vi "HFRR ADV v015 new software.vi"() -> ()   [LabVIEW 2025] (continued)
              frame False {
              }
              frame True {
                n2567 = local write "Rt 3"(FALSE ("Rt 3")) -> ()
                n2568 = local write "Json End Flg"(TRUE ("Upld AR 2")) -> ()
              }
            }
            "Rt" <- TRUE ("Rt")
            "Rt 2" <- FALSE ("Rt")
          }
          frame True {
            n2569 = local read "Rt"() -> (w3002:bool)
            n2570 = local write "Rt 2"(TRUE ("Rt 2")) -> ()
            n2571 = case shown="True" w3002 {
              frame False {
              }
              frame True {
                w3003 = TRUE ("Upld AR 2")
                n2572 = local write "Rt"(FALSE ("Rt")) -> ()
                n2573 = local write "Upld AR"(w3003) -> ()
                n2574 = local write "Json St Flg"(w3003) -> ()
              }
            }
            "Rt 3" <- TRUE ("Rt 3")
          }
        }
        n2575 = case shown="True" w2853 {
          tunnel: [FALSE ("RUN") TRUE ("RUN")] -> w2852
          tunnel: [_ 2] -> w2846
          frame False {
          }
          frame True {
          }
        }
        n2576 = case shown="True" w2851 {
          tunnel: [FALSE ("RUN") TRUE ("RUN")] -> w2850
          tunnel: [_ 3] -> w2845
          frame False {
          }
          frame True {
          }
        }
        n2577 = case shown="\"Acquire\"" w2831 {
          tunnel: w2833 -> [_ w3064]
          frame Default {
            w3063 = 0.0 ("output")
            n2578 = local write "PID-out"(w3063) -> ()
            n2579 = local write "Frequency ( Hz )"(w3063) -> ()
          }
          frame "Acquire" {
            n2580 = stacked-sequence {
              frame #0 {
                n2581 = local read "Auto Start Test"() -> (w3066:bool)
                n2582 = case shown="True" w3066 {
                  tunnel: "RUN" -> [w3087 w3090]
                  tunnel: [w3087 w3089] -> w3067
                  frame False {
                  }
                  frame True {
                    n2583 = local read "Auto Start Temp"() -> (w3088:bool)
                    n2584 = Or(x=w3090, y=w3088) -> (x .or. y?=w3089:bool)
                  }
                }
                n2585 = local read "clk"() -> (w3086:dbl)
                n2586 = local read "Save"() -> (w3082:bool)
                n2587 = Equal?(x=w3086, y=0.0) -> (x = y?=w3083:bool)
                n2588 = And(x=w3083, y=w3082) -> (x .and. y?=w3084:bool)
                n2589 = Not(x="Engage") -> (.not. x?=w3073:bool)
                n2590 = case shown="False" w3067 {
                  tunnel: [0.0 w3113] -> w3069
                  frame False {
                    (unwired) TRUE ("Visible")
                    n2591 = local read "Auto Start Test"() -> (w3094:bool)
                    n2592 = local write "Start Time"(TRUE ("Start Time")) -> ()
                    n2593 = property on="Stroke 2" class="DigNum (strict)"("Visible"=FALSE) -> ()  [unwired: 2 in, 2 out]
                    n2594 = case shown="False" w3094 {
                      frame False {
                        n2595 = property on="Heater Button" class="Bool (strict)"("DisabledEnum"=T18."Enabled" ("Disabled")) -> ()  [unwired: 2 in, 2 out]
                        n2596 = property on="Humidity" class="Bool (strict)"("DisabledEnum"=T18."Enabled" ("Disabled")) -> ()  [unwired: 2 in, 2 out]
                      }
                      frame True {
                      }
                    }
                    n2597 = case shown="False" "TestCompFlg" {
                      frame False {
                        n2598 = local read "StartFlg"() -> (w3102:bool)
                        n2599 = case shown="True" w3102 {
                          frame False {
                          }
                          frame True {
                            n2600 = stacked-sequence {
                              frame #0 {
                                n2601 = local read "EVENT LOG"() -> (w3106:string)
                                n2602 = call "Event Log.vi"("Content"="Test was interrupted", "EVENT LOG"=w3106) -> ("EVENT LOG"=w3107:string)  [unwired: 8 in, 1 out]
                                n2603 = local write "EVENT LOG"(w3107) -> ()
                                n2604 = property on="RUN" class="Bool (strict)"("Visible"=TRUE) -> ()  [unwired: 2 in, 2 out]
                                n2605 = property on="Auto Start Test" class="Bool (strict)"("Visible"=TRUE) -> ()  [unwired: 2 in, 2 out]
                              }
                              frame #1 {
                                w3109 = FALSE ("StartFlg")
                                n2606 = property on="Heater Button" class="Bool (strict)"("Val(Sgnl)"=FALSE ("Value (Signaling)")) -> ()  [unwired: 2 in, 2 out]
                                n2607 = local write "Heater Button"(w3109) -> ()
                                n2608 = local write "StartFlg"(w3109) -> ()
                                n2609 = local write "Humidity"(w3109) -> ()
                              }
                              frame #2 {
                                n2610 = local write "Command"("VC;0" ("Command")) -> ()
                              }
                              frame #3 {
                                n2611 = Wait (ms)(milliseconds to wait=u32 1500) -> ()  [unwired: 1 out]
                              }
                              frame #4 {
                                n2612 = local write "Command"("HE;0" ("Command")) -> ()
                              }
                            }
                          }
                        }
                      }
                      frame True {
                      }
                    }
                    n2613 = local write "String 14"("Test will autostart once parameters reach the set value." ("String 14")) -> ()
                  }
                  frame True {
                    (unwired) FALSE ("Visible")
                    n2614 = property on="Stroke 2" class="DigNum (strict)"("Visible"=TRUE) -> ()  [unwired: 2 in, 2 out]
                    n2615 = property on="STOP 2" class="Bool (strict)"("Disabled"=u8 2) -> ()  [unwired: 2 in, 2 out]
                    n2616 = local write "String 14"(" Running....." ("String 14")) -> ()
                    n2617 = property on="Heater Button" class="Bool (strict)"("DisabledEnum"=T18."Disabled and Grayed Out" ("Disabled")) -> ()  [unwired: 2 in, 2 out]
                    n2618 = property on="Humidity" class="Bool (strict)"("DisabledEnum"=T18."Disabled and Grayed Out" ("Disabled")) -> ()  [unwired: 2 in, 2 out]
                    n2619 = case shown="True" "Start Time" {
                      selector: "Start Time" -> [_ w3132]
                      frame False {
                      }
                      frame True {
                        n2620 = Not(x=w3132) -> (.not. x?=w3131:bool)
                        n2621 = local write "Start Time"(w3131) -> ()
                        n2622 = local read "EVENT LOG"() -> (w3133:string)
                        n2623 = call "Event Log.vi"("Content"="Test in progress", "EVENT LOG"=w3133) -> ("EVENT LOG"=w3135:string)  [unwired: 8 in, 1 out]
                        n2624 = local write "EVENT LOG"(w3135) -> ()
                      }
                    }
                    n2625 = disable-structure shown="Enabled" {
                      disable-tunnel: [w3124 w3130] -> w3113
                      frame Disabled {
                        n2626 = local read "Set Hz"() -> (w3127:dbl)
                        n2627 = call <vilib>:"Uniform White Noise Waveform.vi"() -> ("signal out"=w3126:waveform(dbl))  [unwired: 10 in, 1 out]
                        n2628 = Random Number (0-1)() -> (number: 0 to 1=w3123:dbl)
                        n2629 = Add(x=w3127, y=w3126) -> (x+y=w3125:waveform(dbl))
                        n2630 = Multiply(x=ext 0.01 ("y"), y=w3123) -> (x*y=w3121:ext)
                        n2631 = Multiply(x=w3125, y=w3121) -> (x*y=w3124:waveform(ext))
                      }
                      frame Enabled {
                        n2632 = call-poly <vilib>:"Random Number (Range).vi"("lower bound (0)"=49.89, "upper bound (100)"=50.8) -> ("number"=w3130:dbl)  [unwired: 9 in]
                      }
                    }
                    "StartFlg" <- TRUE ("StartFlg")
                  }
                }
                n2633 = case shown="True" w3084 {
                  frame False {
                  }
                  frame True {
                    n2634 = local write "clk"(10.0 ("clk")) -> ()
                    n2635 = Get Date/Time In Seconds() -> (seconds since 1Jan1904=w3138:timestamp)
                    n2636 = To Double Precision Float(number=w3138) -> (double precision float=w3136:dbl)
                    n2637 = local write "acq timer"(w3136) -> ()
                    n2638 = local write "act save time"(w3136) -> ()
                  }
                }
                n2639 = call "Elapsed Time"("Time Target (s)"="Countdown", "Reset"=w3073) -> ("Elapsed Time (s)"=w3078:dbl, "Time has Elapsed"=w3076:bool)  [unwired: 10 in, 6 out]
                "Countdown 2" <- w3078
                n2640 = Subtract(x=w3078, y=2.0) -> (x-y=w3081:dbl)
                n2641 = Less?(x=w3081, y="Countdown") -> (x < y?=w3079:bool)
                n2642 = And(x=w3079, y=w3076) -> (x .and. y?=w3075:bool)
                n2643 = case shown="True" w3075 {
                  frame False {
                  }
                  frame True {
                    (unwired) dbl[] [] ("History Data")
                    n2644 = local write "Engage"(FALSE ("Engage")) -> ()
                    n2645 = local write "RUN"(TRUE ("RUN")) -> ()
                    n2646 = local read "Humidity ( %RH )"() -> (→"Rh Before":dbl)
                  }
                }
                n2647 = local read "Test \nStatus"() -> (w3071:bool)
                n2648 = Select(t=w3069, s=w3071, f=0.0) -> (s? t:f=w3070:dbl)
                n2649 = local write "Frequency ( Hz )"(w3070) -> ()
              }
              frame #1 {
                w3161 = 1000000.0 ("x")
                # "HC;1/0\nST;VALUE"
                # "Elapsed time\ncof\nstroke\nAir temp\nTemp\nHumidity"
                # "acq timer\n\nact save time"
                # "convert to microseconds"
                n2650 = local read "COUNT"() -> (w3144:i32)
                n2651 = local read "Rate"() -> (w3157:dbl)
                n2652 = Divide(x=w3161, y=w3157) -> (x/y=w3162:dbl)
                n2653 = Greater Or Equal?(x=w3144, y=250) -> (x >= y?=w3143:bool)
                n2654 = Get Date/Time In Seconds() -> (seconds since 1Jan1904=w3164:timestamp)
                n2655 = case shown="True" w3143 {
                  frame False {
                    n2656 = local read "COUNT"() -> (w3165:i32)
                    n2657 = Increment(x=w3165) -> (x+1=w3166:i32)
                    n2658 = local write "COUNT"(w3166) -> ()
                  }
                  frame True {
                    n2659 = local write "COUNT"(0 ("COUNT")) -> ()
                  }
                }
                n2660 = local read "Samplingtime 2"() -> (w3142:dbl)
                n2661 = local read "act save time"() -> (w3159:dbl)
                n2662 = Divide(x=w3162, y=w3161) -> (x/y=w3160:dbl)
                n2663 = To Double Precision Float(number=w3164) -> (double precision float=w3153:dbl)
                n2664 = Add(x=w3159, y=w3142) -> (x+y=w3158:dbl)
                n2665 = local read "acq timer"() -> (w3163:dbl)
                n2666 = local read "COUNT"() -> (w3146:i32)
                n2667 = Greater Or Equal?(x=w3153, y=w3158) -> (x >= y?=w3141:bool)
                n2668 = Multiply(x=w3160, y=w3146) -> (x*y=w3152:dbl)
                n2669 = Subtract(x=w3153, y=w3163) -> (x-y=w3155:dbl)
                n2670 = local read "Save"() -> (w3156:bool)
                n2671 = Add(x=w3155, y=w3152) -> (x+y=w3139:dbl)
                "Elapsed time 3" <- w3139
                n2672 = And(x=w3141, y=w3156) -> (x .and. y?=w3154:bool)
                n2673 = Divide(x=w3139, y=60.0) -> (x/y=w3150:dbl)
                n2674 = local read "Test \nStatus"() -> (w3140:bool)
                n2675 = local read "clk"() -> (w3147:dbl)
                n2676 = Equal?(x=w3147, y=10.0) -> (x = y?=w3149:bool)
                n2677 = case shown="True" w3154 {
                  tunnel: w3153 -> [_ w3277]
                  tunnel: [FALSE ("Boolean 2") TRUE ("Boolean 2")] -> _
                  frame False {
                  }
                  frame True {
                    w3231 = ";" ("Substring")
                    # "Pid out/\nFreq response value"
                    n2678 = local write "act save time"(w3277) -> ()
                    n2679 = local read "FILE"() -> (w3225:string)
                    n2680 = call "file check.vi"("file name in"=w3225) -> ("error out"=w3228:errorcluster, "file name out"=w3223:string)  [unwired: 9 in]
                    n2681 = local read "LVDT STROKE"() -> (w3220:dbl)
                    n2682 = local read "Add up Stroke"() -> (w3218:dbl)
                    n2683 = call "FILE PATH CREATION.vi"("error in"=w3228, "FILE NAME :"=w3223) -> ("FILE OUT"=w3226:path)  [unwired: 8 in, 1 out]
                    n2684 = Concatenate Strings(w3223, ".dgf" ("Substring")) -> (w3227:string)
                    n2685 = Subtract(x=w3220, y=w3218) -> (x-y=w3219:dbl)
                    n2686 = Absolute Value(x=w3219) -> (abs(x)=w3217:dbl)
                    n2687 = local read "FF 2"() -> (→"Frictional Force ( N )" →"Frictional Force ( N )":dbl)
                    n2688 = Build Path(base path=w3226, name or relative path=w3227) -> (appended path=w3222:path)
                    n2689 = local read "COF 2"() -> (w3236:dbl)
                    "cof" <- w3236
                    "Coefficient of Friction" <- w3236
                    "COF 4" <- w3236
                    "Coefficient of Friction" <- w3236
                    n2690 = local read "TEMP"() -> (w3239:dbl)
                    "Temp" <- w3239
                    "Temperature ( Deg C )" <- w3239
                    n2691 = local read "Humidity ( %RH )"() -> (w3238:dbl)
                    "Humidity ( %RH )" <- w3238
                    "Humidity ( %RH )" <- w3238
                    n2692 = local read "Frequency ( Hz )"() -> (w3245:dbl)
                    n2693 = call <vilib>:"Mean PtByPt.vi"("x"=w3217, "sample length"="STROKE FILTER") -> ("mean"=w3216:dbl)  [unwired: 2 in, 1 out]
                    n2694 = local read "Elapsed time"() -> (w3270:dbl)
                    n2695 = local read "AIR TEMP"() -> (w3243:dbl)
                    n2696 = local read "PID-out"() -> (w3248:dbl)
                    n2697 = local write "Temperature ( Deg C )"(w3239) -> ()
                    n2698 = Number To Fractional String(number=w3216, width (-)=i16 9 ("precision (6)"), precision (6)=i16 6) -> (F-format string=w3263:string)  [unwired: 1 in]
                    n2699 = Number To Fractional String(number=w3243, width (-)=i16 9 ("precision (6)"), precision (6)=i16 3) -> (F-format string=w3262:string)  [unwired: 1 in]
                    n2700 = Number To Fractional String(number=w3239, width (-)=i16 9 ("precision (6)"), precision (6)=i16 3) -> (F-format string=w3259:string)  [unwired: 1 in]
                    n2701 = Number To Fractional String(number=w3238, width (-)=i16 9 ("precision (6)"), precision (6)=i16 3) -> (F-format string=w3256:string)  [unwired: 1 in]
                    n2702 = Number To Fractional String(number=0.0, width (-)=i16 9 ("precision (6)"), precision (6)=i16 3) -> (F-format string=w3253:string)  [unwired: 1 in]
                    n2703 = Number To Fractional String(number=w3248, width (-)=i16 9 ("precision (6)"), precision (6)=i16 3) -> (F-format string=w3249:string)  [unwired: 1 in]
                    n2704 = Number To Fractional String(number=w3245, width (-)=i16 9 ("precision (6)"), precision (6)=i16 3) -> (F-format string=w3244:string)  [unwired: 1 in]
                    n2705 = Number To Fractional String(number=w3236, width (-)=i16 9 ("precision (6)"), precision (6)=i16 6) -> (F-format string=w3271:string)  [unwired: 1 in]
                    n2706 = Number To Fractional String(number=w3270, width (-)=i16 14 ("precision (6)"), precision (6)=i16 3) -> (F-format string=w3272:string)  [unwired: 1 in]
                    n2707 = Bundle("y"=1.02, "mean"=w3216, "y"=0.98) -> (w3237:cluster{"y":dbl, "mean":dbl, "y":dbl})  [unwired: 1 in]
                    n2708 = Number To Fractional String(number="Ambient Humidity :", width (-)=i16 9 ("precision (6)"), precision (6)=i16 6) -> (F-format string=w3229:string)  [unwired: 1 in]
                    n2709 = local read "RUN"() -> (w3235:bool)
                    n2710 = case shown="True" w3235 {
                      tunnel: w3237 -> [_ w3282]
                      tunnel: w3216 -> [_ w3281]
                      tunnel: w3216 -> [_ w3279]
                      tunnel: w3216 -> [_ w3280]
                      frame False {
                      }
                      frame True {
                        "Stroke ( mm )" <- w3282
                        "Stroke ( mm )" <- w3282
                        "Stroke 4" <- w3281
                        "Stroke 3" <- w3279
                        "Stroke 2" <- w3280
                        "measured_stroke" <- w3279
                      }
                    }
                    n2711 = Concatenate Strings(w3272, w3231, w3271, w3231, w3263, w3231, w3262, w3231, w3259, w3231, w3256, w3231, w3253, w3231, w3249, w3231, w3244, w3231, w3229, "\r") -> (w3269:string)
                    n2712 = call <vilib>:"Write Characters To File.vi"("append to file? (new file:F)"=TRUE, "character string"=w3269, "file path (dialog if empty)"=w3222) -> ()  [unwired: 2 in, 1 out]
                    "refresh flag" <- TRUE ("refresh flag")
                  }
                }
                n2713 = case shown="True" w3140 {
                  tunnel: w3150 -> [_ w3176]
                  tunnel: w3155 -> [_ w3186]
                  tunnel: [0.0 w3182] -> _
                  tunnel: w3149 -> [_ w3181]
                  tunnel: [0.0 w3180] -> _
                  tunnel: w3139 -> [_ w3180]
                  tunnel: w3153 -> [w3169 _]
                  frame False {
                    n2714 = local write "acq timer"(w3169) -> ()
                    n2715 = local write "Test Duration Status"(0.0 ("Test Duration Status")) -> ()
                  }
                  frame True {
                    n2716 = local read "Set Hz"() -> (w3183:dbl)
                    n2717 = local write "Elapsed time"(w3176) -> ()
                    n2718 = local read "test time"() -> (w3175:dbl)
                    n2719 = Multiply(x=w3186, y=w3183) -> (x*y=w3185:dbl)
                    n2720 = case shown="False" w3181 {
                      tunnel: w3185 -> [w3187 _]
                      tunnel: [w3187 1.0] -> w3182
                      frame False {
                        n2721 = local write "Cycles elapsed"(w3187) -> ()
                      }
                      frame True {
                      }
                    }
                    n2722 = Greater?(x=w3176, y=w3175) -> (0:w3184:bool)
                    n2723 = Subtract(x=w3175, y=w3176) -> (x-y=w3174:dbl)
                    "time" <- w3174
                    n2724 = Multiply(x=w3174, y=60.0) -> (x*y=w3173:dbl)
                    n2725 = local write "Time Remaining"(w3173) -> ()
                    n2726 = local write "Remaining Time"(w3173) -> ()
                    n2727 = case shown="True" w3184 {
                      frame False {
                      }
                      frame True {
                        n2728 = stacked-sequence {
                          frame #0 {
                            w3192 = T18."Enabled" ("Disabled")
                            w3191 = FALSE ("TEST FILE NAM,E SAVED")
                            w3193 = "" ("FILE")
                            w3194 = TRUE ("Visible")
                            n2729 = local write "Humidity"(FALSE ("Humidity")) -> ()
                            n2730 = local write "RUN"(FALSE ("OK Button 2")) -> ()
                            n2731 = local write "Heater Button"(FALSE ("Heater Button")) -> ()
                            n2732 = local write "Auto Start Test"(FALSE ("Auto Start Test")) -> ()
                            n2733 = local write "TestCompFlg"(TRUE ("StpFlg")) -> ()
                            n2734 = local read "Humidity ( %RH )"() -> (→"Rh After":dbl)
                            n2735 = property on="STOP 2" class="Bool (strict)"("Disabled"=u8 0) -> ()  [unwired: 2 in, 2 out]
                            n2736 = local read "EVENT LOG"() -> (w3199:string)
                            n2737 = call "Event Log.vi"("Content"="Test Completed", "EVENT LOG"=w3199) -> ("EVENT LOG"=w3198:string)  [unwired: 8 in, 1 out]
                            n2738 = property on="RUN" class="Bool (strict)"("Visible"=w3194) -> ()  [unwired: 2 in, 2 out]
                            n2739 = property on="Auto Start Test" class="Bool (strict)"("Visible"=w3194) -> ()  [unwired: 2 in, 2 out]
                            n2740 = local write "Batch Ref Num :"(w3193) -> ()
                            n2741 = local write "FILE"(w3193) -> ()
                            n2742 = local write "EVENT LOG"(w3198) -> ()
                            n2743 = local write "TEST FILE NAM,E SAVED"(w3191) -> ()
                            n2744 = local write "Fuel Discription :"(w3193) -> ()
                            n2745 = local write "START TEMP"(w3191) -> ()
                            n2746 = local write "Remarks :"(w3193) -> ()
                            n2747 = local write "Main Dashboard Buttons"(T1."Imaging" ("Main Dashboard Buttons")) -> ()
                            n2748 = local write "Main Tab"(T2."Adv Scar" ("Main Tab")) -> ()
                            n2749 = property on="FRICVALZ 2" class="Bool (strict)"("DisabledEnum"=w3192) -> ()  [unwired: 2 in, 2 out]
                            n2750 = property on="FRICVALZ 3" class="Bool (strict)"("DisabledEnum"=w3192) -> ()  [unwired: 2 in, 2 out]
                            n2751 = property on="FRICVALZ 4" class="Bool (strict)"("DisabledEnum"=w3192) -> ()  [unwired: 2 in, 2 out]
                          }
                          frame #1 {
                            n2752 = Wait (ms)(milliseconds to wait=u32 1500) -> ()  [unwired: 1 out]
                          }
                          frame #2 {
                            n2753 = local write "Command"("VC;0") -> ()
                          }
                          frame #3 {
                            n2754 = Wait (ms)(milliseconds to wait=u32 1500) -> ()  [unwired: 1 out]
                          }
                          frame #4 {
                            n2755 = local write "Command"("VC;0") -> ()
                          }
                          frame #5 {
                            n2756 = Wait (ms)(milliseconds to wait=u32 1500) -> ()  [unwired: 1 out]
                          }
                          frame #6 {
                            n2757 = local write "Command"("ST;0") -> ()
                          }
                          frame #7 {
                            n2758 = local write "measured_stroke"(0.0 ("measured_stroke")) -> ()
                            n2759 = Wait (ms)(milliseconds to wait=u32 1500) -> ()  [unwired: 1 out]
                          }
                          frame #8 {
                            n2760 = local write "Command"("HE;0") -> ()
                          }
                        }
                      }
                    }
                    n2761 = Divide(x=w3176, y=w3175) -> (x/y=w3179:dbl)
                    n2762 = Multiply(x=w3179, y=100.0) -> (x*y=w3177:dbl)
                    n2763 = local write "Test Duration Status"(w3177) -> ()
                  }
                }
              }
              frame #2 {
                n2764 = case shown="True" "Heater Button" {
                  tunnel: [0.0 ("output") w3305] -> w3283
                  frame False {
                    w3286 = TRUE ("tmpchk")
                    n2765 = local read "TEMP"() -> (w3287:dbl)
                    n2766 = local write "Temp ini"(w3287) -> ()
                    n2767 = local write "Reset 4"(w3286) -> ()
                    n2768 = local write "tmpchk"(w3286) -> ()
                    n2769 = local write "reinit"(TRUE ("reinit")) -> ()
                    n2770 = local write "manual temp log"(TRUE ("manual temp log")) -> ()
                  }
                  frame True {
                    # "Logic to turn off\nthe heater when \ntemp is not rising.\nTime - 60 sec\nDelta t- 5°c"
                    n2771 = local read "Temp ini"() -> (w3294:dbl)
                    n2772 = local read "Auto Start Test"() -> (w3290:bool)
                    n2773 = Less?(x=w3294, y=53.0) -> (x < y?=w3292:bool)
                    n2774 = case shown="False" w3290 {
                      frame False {
                        n2775 = local read "Set Temp"() -> (w3314:dbl)
                        n2776 = local read "TEMP"() -> (w3313:dbl)
                        n2777 = Subtract(x=w3314, y=w3313) -> (x-y=w3312:dbl)
                        n2778 = Absolute Value(x=w3312) -> (abs(x)=w3311:dbl)
                        n2779 = Less?(x=w3311, y=0.5) -> (x < y?=w3309:bool)
                        n2780 = case shown="True" w3309 {
                          tunnel: "manual temp log" -> [_ w3315]
                          frame False {
                          }
                          frame True {
                            n2781 = case shown="True" w3315 {
                              selector: w3315 -> [_ w3316]
                              frame False {
                              }
                              frame True {
                                # "#Event log"
                                n2782 = Not(x=w3316) -> (.not. x?=w3317:bool)
                                n2783 = local write "manual temp log"(w3317) -> ()
                                n2784 = local read "EVENT LOG"() -> (w3320:string)
                                n2785 = call "Event Log.vi"("Content"="Target Temperature reached", "EVENT LOG"=w3320) -> ("EVENT LOG"=w3319:string)  [unwired: 8 in, 1 out]
                                n2786 = local write "EVENT LOG"(w3319) -> ()
                              }
                            }
                          }
                        }
                      }
                      frame True {
                        n2787 = local write "manual temp log"(TRUE ("manual temp log")) -> ()
                      }
                    }
                    n2788 = And(x="tmpchk", y=w3292) -> (x .and. y?=w3295:bool)
                    n2789 = case shown="True" w3295 {
                      frame False {
                      }
                      frame True {
                        n2790 = call "Elapsed Time8"("Time Target (s)"=300.0, "Reset"="Reset 4") -> ("Time has Elapsed"=w3322:bool)  [unwired: 10 in, 7 out]
                        n2791 = flat-sequence {
                          tunnel: w3322 -> [_]
                          frame #0 {
                            n2792 = local write "Reset 4"(FALSE ("Reset 4")) -> ()
                          }
                        }
                        n2793 = case shown="True" w3322 {
                          frame False {
                          }
                          frame True {
                            n2794 = local read "Temp ini"() -> (w3329:dbl)
                            n2795 = Add(x=w3329, y=5.0) -> (x+y=w3327:dbl)
                            n2796 = local read "TEMP"() -> (w3330:dbl)
                            n2797 = Greater?(x=w3330, y=w3327) -> (0:w3328:bool)
                            n2798 = case shown="False" w3328 {
                              frame False {
                                n2799 = local write "Heater Button"(FALSE ("Heater Button")) -> ()
                              }
                              frame True {
                                n2800 = local write "tmpchk"(FALSE ("tmpchk")) -> ()
                              }
                            }
                          }
                        }
                      }
                    }
                    n2801 = local read "Set Temp"() -> (w3303:dbl)
                    n2802 = local read "TEMP"() -> (w3297:dbl)
                    n2803 = call-poly <vilib>:"PID.vi"("reinitialize? (F)"="reinit", "dt (s)"=-1.0, "process variable"=w3297, "setpoint"=w3303) -> ("output"=w3300:dbl)  [unwired: 6 in, 1 out]
                    n2804 = Subtract(x=w3303, y=w3297) -> (x-y=w3304:dbl)
                    n2805 = Add(x=w3303, y=0.5) -> (x+y=w3301:dbl)
                    n2806 = Greater Or Equal?(x=w3297, y=w3301) -> ()  [unwired: 1 out]
                    n2807 = Select(t=0.0, s=FALSE, f=w3300) -> (s? t:f=w3299:dbl)
                    "PID output" <- w3299
                    n2808 = flat-sequence {
                      tunnel: w3299 -> [w3333]
                      tunnel: [w3333] -> w3305
                      frame #0 {
                        n2809 = local write "reinit"(FALSE ("reinit")) -> ()
                      }
                    }
                    n2810 = Bundle(w3304, "output"=w3299, "TEMP"=w3297) -> ()  [unwired: 1 in, 1 out]
                  }
                }
                "PID-out" <- w3283
              }
              frame #3 {
                n2811 = local read "TEMP"() -> (w3335:dbl)
                n2812 = Greater Or Equal?(x=w3335, y="Set Temp 2") -> (x >= y?=w3340:bool)
                n2813 = case shown="True" w3340 {
                  tunnel: [FALSE TRUE] -> w3338
                  frame False {
                  }
                  frame True {
                  }
                }
                "Status 13" <- w3338
                n2814 = And(x=w3338, y="trip1 8") -> (x .and. y?=w3337:bool)
                n2815 = case shown="True" w3337 {
                  frame False {
                    n2816 = local write "Heater Trip Temp"(TRUE ("Heater Trip Temp")) -> ()
                  }
                  frame True {
                    w3343 = FALSE ("OK Button 2")
                    n2817 = case shown="True" "Heater Trip Temp" {
                      selector: "Heater Trip Temp" -> [_ w3345]
                      frame False {
                      }
                      frame True {
                        n2818 = Not(x=w3345) -> (.not. x?=w3344:bool)
                        n2819 = local read "EVENT LOG"() -> (w3348:string)
                        n2820 = local write "Heater Trip Temp"(w3344) -> ()
                        n2821 = call "Event Log.vi"("Content"="Heater Trip", "EVENT LOG"=w3348) -> ("EVENT LOG"=w3347:string)  [unwired: 8 in, 1 out]
                        n2822 = local write "EVENT LOG"(w3347) -> ()
                      }
                    }
                    n2823 = local write "RUN"(w3343) -> ()
                    n2824 = property on="Auto Start Test" class="Bool (strict)"("Value"=w3343) -> ()  [unwired: 2 in, 2 out]
                    n2825 = local write "Heater Button"(w3343) -> ()
                  }
                }
              }
            }
            n2826 = case shown="False" w3064 {
              frame False {
                n2827 = disable-structure shown="Disabled" {
                  frame Disabled {
                    n2828 = stacked-sequence {
                      frame #0 {
                        n2829 = local write "RUN"(FALSE ("OK Button 2")) -> ()
                      }
                      frame #1 {
                      }
                    }
                  }
                  frame Enabled {
                  }
                }
              }
              frame True {
              }
            }
          }
        }
        n2830 = local read "airtempflg"() -> (w2856:bool)
        n2831 = Or(x=w2856, y=w2854) -> (x .or. y?=w2857:bool)
        n2832 = Insert Into Array(array=string[] ["Air Temperature has reached set value,", "Humidity has reached set value,", "Sample Temperaturehas reached set value,", ""], index=0, new element="") -> (w2842:string[])
        n2833 = Build Array(w2847, w2846, w2845) -> (w2843:i32[])
        n2834 = disable-structure shown="Disabled" {
          disable-tunnel: w2857 -> [w2934 _]
          disable-tunnel: w2852 -> [w2933 _]
          disable-tunnel: w2850 -> [w2932 _]
          frame Disabled {
            n2835 = Compound Arithmetic op=AND(w2934, w2933, w2932) -> ()  [unwired: 1 out]
            n2836 = case shown="True" {
              selector: _ -> [_ _]
              frame False {
              }
              frame True {
                w2935 = FALSE ("autostrtflg")
                n2837 = local write "RUN"(TRUE ("RUN")) -> ()
                n2838 = local write "autostrtflg"(w2935) -> ()
                n2839 = local write "autostart"(w2935) -> ()
                n2840 = local write "String 14"(" Running....." ("String 14")) -> ()
              }
            }
          }
          frame Enabled {
          }
        }
        n2841 = for {
          tunnel: w2843 -> [w2985] mode=indexing
          tunnel: w2842 -> [w2984]
          shift-right: [w2981] -> w2841
          shift-left: "" -> [w2983]
          n2842 = Index Array(array=w2984, index=w2985) -> (element=w2982:string)
          n2843 = Concatenate Strings(w2982, w2983) -> (w2981:string)
        }
        n2844 = local write "autostart 2"(w2841) -> ()
        n2845 = local read "Reset Graph"() -> (w2830:bool)
        n2846 = case shown="True" w2830 {
          selector: w2830 -> [_ w2884]
          frame False {
          }
          frame True {
            w2898 = 0.0 ("X Scale.Range:Maximum")
            n2847 = Not(x=w2884) -> (.not. x?=w2883:bool)
            n2848 = local write "Reset Graph"(w2883) -> ()
            n2849 = property on="Electrical Contact Resistance ( % )" class="WFChart (strict)"("XScale.Maximum"=600.0 ("X Scale.Range:Maximum"), "XScale.Minimum"=0.0 ("X Scale.Range:Minimum"), "YScale.Maximum"=100.0 ("Y Scale.Range:Maximum"), "YScale.Minimum"=0.0 ("Y Scale.Range:Minimum")) -> ()  [unwired: 2 in, 2 out]
            n2850 = property on="Frictional Force ( N )" class="WFChart (strict)"("XScale.Maximum"=600.0 ("X Scale.Range:Maximum"), "XScale.Minimum"=0.0 ("X Scale.Range:Minimum"), "YScale.Maximum"=100.0 ("Y Scale.Range:Maximum"), "YScale.Minimum"=0.0 ("Y Scale.Range:Minimum")) -> ()  [unwired: 2 in, 2 out]
            n2851 = property on="Temperature ( Deg C )" class="WFChart (strict)"("XScale.Maximum"=600.0 ("X Scale.Range:Maximum"), "XScale.Minimum"=0.0 ("X Scale.Range:Minimum"), "YScale.Maximum"=100.0 ("Y Scale.Range:Maximum"), "YScale.Minimum"=0.0 ("Y Scale.Range:Minimum")) -> ()  [unwired: 2 in, 2 out]
            n2852 = property on="Humidity ( %RH )" class="WFChart (strict)"("XScale.Maximum"=600.0 ("X Scale.Range:Maximum"), "XScale.Minimum"=0.0 ("X Scale.Range:Minimum"), "YScale.Maximum"=100.0 ("Y Scale.Range:Maximum"), "YScale.Minimum"=0.0 ("Y Scale.Range:Minimum")) -> ()  [unwired: 2 in, 2 out]
            n2853 = property on="Stroke ( mm )" class="WFChart (strict)"("XScale.Maximum"=600.0 ("X Scale.Range:Maximum"), "XScale.Minimum"=0.0 ("X Scale.Range:Minimum"), "YScale.Maximum"=100.0 ("Y Scale.Range:Maximum"), "YScale.Minimum"=0.0 ("Y Scale.Range:Minimum")) -> ()  [unwired: 2 in, 2 out]
            n2854 = property on="Coefficient of Friction" class="WFChart (strict)"("XScale.Maximum"=600.0 ("X Scale.Range:Maximum"), "XScale.Minimum"=0.0 ("X Scale.Range:Minimum"), "YScale.Maximum"=100.0 ("Y Scale.Range:Maximum"), "YScale.Minimum"=0.0 ("Y Scale.Range:Minimum")) -> ()  [unwired: 2 in, 2 out]
            n2855 = property on="Electrical Contact Resistance ( % )" class="WFChart (strict)"("XScale.Minimum"=0.0 ("X Scale.Range:Minimum"), "XScale.Maximum"=600.0 ("X Scale.Range:Maximum"), "YScale.Minimum"=0.0 ("Y Scale.Range:Minimum"), "YScale.Maximum"=100.0 ("Y Scale.Range:Maximum")) -> ()  [unwired: 2 in, 2 out]
            n2856 = property on="Temperature ( Deg C )" class="WFChart (strict)"("XScale.Minimum"=0.0 ("X Scale.Range:Minimum"), "XScale.Maximum"=600.0 ("X Scale.Range:Maximum"), "YScale.Minimum"=0.0 ("Y Scale.Range:Minimum"), "YScale.Maximum"=100.0 ("Y Scale.Range:Maximum")) -> ()  [unwired: 2 in, 2 out]
            n2857 = property on="Coefficient of Friction" class="WFChart (strict)"("XScale.Minimum"=0.0 ("X Scale.Range:Minimum"), "XScale.Maximum"=600.0 ("X Scale.Range:Maximum"), "YScale.Maximum"=1.0 ("X Scale.Range:Minimum"), "YScale.Minimum"=0.0 ("X Scale.Range:Minimum")) -> ()  [unwired: 2 in, 2 out]
            n2858 = property on="Frictional Force ( N )" class="WFChart (strict)"("XScale.Maximum"=600.0 ("X Scale.Range:Maximum"), "XScale.Minimum"=w2898, "YScale.Maximum"=10.0 ("Y Scale.Range:Maximum"), "YScale.Minimum"=w2898) -> ()  [unwired: 2 in, 2 out]
            n2859 = property on="Stroke ( mm )" class="WFChart (strict)"("XScale.Maximum"=600.0 ("X Scale.Range:Maximum"), "XScale.Minimum"=0.0 ("X Scale.Range:Minimum"), "YScale.Maximum"=100.0 ("Y Scale.Range:Maximum"), "YScale.Minimum"=0.0 ("Y Scale.Range:Minimum")) -> ()  [unwired: 2 in, 2 out]
            n2860 = property on="Humidity ( %RH )" class="WFChart (strict)"("XScale.Maximum"=600.0 ("X Scale.Range:Maximum"), "XScale.Minimum"=0.0 ("X Scale.Range:Minimum"), "YScale.Maximum"=100.0 ("Y Scale.Range:Maximum"), "YScale.Minimum"=0.0 ("Y Scale.Range:Minimum")) -> ()  [unwired: 2 in, 2 out]
          }
        }
      }
      frame "Compare Files" {
        # "Elapsed time\ncof\nstroke\nAir temp\nTemp\nHumidity"
        n2861 = case shown="True" "RSTV1 2" {
          frame False {
          }
          frame True {
            n2862 = property on="Humidity ( %RH )" class="XYGraph (strict)"("Y Scale.Display Format:Precision"=u8 0 ("Y Scale.Format & Precision:Precision")) -> ()  [unwired: 2 in, 2 out]
            n2863 = property on="Humidity ( %RH )" class="XYGraph (strict)"("X Scale.Range:Minimum"=0.0, "X Scale.Range:Maximum"=75.0, "Y Scale.Range:Minimum"=48.0, "Y Scale.Range:Maximum"=58.0) -> ()  [unwired: 2 in, 2 out]
          }
        }
        n2864 = case shown="True" "RST CP 2" {
          frame False {
          }
          frame True {
            n2865 = property on="XY Graph 13" class="XYGraph (strict)"("Y Scale.Display Format:Precision"=u8 0 ("Y Scale.Format & Precision:Precision")) -> ()  [unwired: 2 in, 2 out]
            n2866 = property on="XY Graph 13" class="XYGraph (strict)"("X Scale.Range:Minimum"=0.0, "X Scale.Range:Maximum"=75.0, "Y Scale.Range:Minimum"=0.0, "Y Scale.Range:Maximum"=100.0) -> ()  [unwired: 2 in, 2 out]
          }
        }
        n2867 = case shown="True" "RST CP" {
          frame False {
          }
          frame True {
            n2868 = property on="Sample Temperature ( °C )" class="XYGraph (strict)"("Y Scale.Display Format:Precision"=u8 2 ("Y Scale.Format & Precision:Precision")) -> ()  [unwired: 2 in, 2 out]
            n2869 = property on="Sample Temperature ( °C )" class="XYGraph (strict)"("X Scale.Range:Minimum"=0.0, "X Scale.Range:Maximum"=75.0, "Y Scale.Range:Minimum"=58.0, "Y Scale.Range:Maximum"=62.0) -> ()  [unwired: 2 in, 2 out]
          }
        }
        n2870 = case shown="True" "RSTV1 3" {
          frame False {
          }
          frame True {
            n2871 = property on="Air Temperature  ( °C )" class="XYGraph (strict)"("Y Scale.Display Format:Precision"=u8 2 ("Y Scale.Format & Precision:Precision")) -> ()  [unwired: 2 in, 2 out]
            n2872 = property on="Air Temperature  ( °C )" class="XYGraph (strict)"("X Scale.Range:Minimum"=0.0 ("Y Scale.Range:Minimum"), "X Scale.Range:Maximum"=75.0 ("Y Scale.Range:Maximum"), "Y Scale.Range:Minimum"=20.0 ("X Scale.Range:Minimum"), "Y Scale.Range:Maximum"=26.0 ("X Scale.Range:Maximum")) -> ()  [unwired: 2 in, 2 out]
          }
        }
        n2873 = case shown="True" "RSTV1 4" {
          frame False {
          }
          frame True {
            n2874 = property on="Stroke ( mm )" class="XYGraph (strict)"("Y Scale.Display Format:Precision"=u8 2 ("Y Scale.Format & Precision:Precision")) -> ()  [unwired: 2 in, 2 out]
            n2875 = property on="Stroke ( mm )" class="XYGraph (strict)"("X Scale.Range:Minimum"=0.0 ("Y Scale.Range:Maximum"), "X Scale.Range:Maximum"=75.0 ("X Scale.Range:Minimum"), "Y Scale.Range:Minimum"=0.98, "Y Scale.Range:Maximum"=1.02) -> ()  [unwired: 2 in, 2 out]
          }
        }
        n2876 = case shown="True" "rstv2" {
          frame False {
          }
          frame True {
            n2877 = property on="Coefficient Of Friction" class="XYGraph (strict)"("Y Scale.Display Format:Precision"=u8 3 ("Y Scale.Format & Precision:Precision")) -> ()  [unwired: 2 in, 2 out]
            n2878 = property on="Coefficient Of Friction" class="XYGraph (strict)"("X Scale.Range:Minimum"=0.0 ("Y Scale.Range:Maximum"), "X Scale.Range:Maximum"=75.0, "Y Scale.Range:Minimum"=0.0, "Y Scale.Range:Maximum"=1.0 ("X Scale.Range:Minimum")) -> ()  [unwired: 2 in, 2 out]
          }
        }
        n2879 = case shown="True" "RST CP 3" {
          frame False {
          }
          frame True {
            n2880 = property on="Air Temp ( °C ) vs Humidity ( % RH )" class="XYGraph (strict)"("X Scale.Range:Minimum"=18.0, "X Scale.Range:Maximum"=28.0 ("X Scale.Range:Minimum"), "Y Scale.Range:Minimum"=30.0 ("X Scale.Range:Minimum"), "Y Scale.Range:Maximum"=70.0 ("X Scale.Range:Minimum")) -> ()  [unwired: 2 in, 2 out]
          }
        }
        n2881 = case shown="True" "OPEN 1" {
          frame False {
          }
          frame True {
            (unwired) 0  # existing file
            w3624 = "Choose a datalog file to open"  # prompt
            n2882 = local write "OPEN 1"(FALSE ("OPEN 1")) -> ()
            n2883 = String To Path(string="C:\\LAB-IQ\\Data\\") -> (path=w3609:path)
            n2884 = File Dialog(6:"*.dgf" ("pattern"), 7:w3624, 11:w3609) -> (0:w3607:errorcluster, 3:w3615:path)  [unwired: 4 in, 2 out]
            n2885 = Unbundle(w3607) -> ()  [unwired: 3 out]
            n2886 = Strip Path(path=w3615) -> (name=w3614:string)  [unwired: 1 out]
            n2887 = Path To String(path=w3615) -> (string=w3610:string)
            "string1" <- w3610
            n2888 = Match Pattern(string=w3614, regular expression=".dgf") -> (before substring=→"String Control":string)  [unwired: 1 in, 3 out]
            n2889 = Match Pattern(string=w3610, regular expression=".dgf" ("substring (\"\")")) -> (before substring=w3620:string)  [unwired: 1 in, 3 out]
            n2890 = Concatenate Strings(w3620, ".duf" ("Substring")) -> (w3616:string)
            n2891 = String To Path(string=w3616) -> (path=w3621:path)
            n2892 = call <vilib>:"Read Characters From File.vi"("file path (dialog if empty)"=w3621, "start of read offset (chars.:0)"=60 ("start of read offset (chars.: 0)")) -> ("character string"=→"String Control 2":string)  [unwired: 4 in, 3 out]
          }
        }
        n2893 = case shown="True" "OPEN 2" {
          frame False {
          }
          frame True {
            (unwired) 0  # existing file
            w3642 = "Choose a datalog file to open"  # prompt
            n2894 = local write "OPEN 2"(FALSE ("OPEN 1")) -> ()
            n2895 = String To Path(string="C:\\LAB-IQ\\Data\\") -> (path=w3627:path)
            n2896 = File Dialog(6:"*.dgf" ("pattern"), 7:w3642, 11:w3627) -> (0:w3625:errorcluster, 3:w3633:path)  [unwired: 4 in, 2 out]
            n2897 = Unbundle(w3625) -> ()  [unwired: 3 out]
            n2898 = Strip Path(path=w3633) -> (name=w3631:string)  [unwired: 1 out]
            n2899 = Path To String(path=w3633) -> (string=w3628:string)
            "string1 2" <- w3628
            n2900 = Match Pattern(string=w3631, regular expression=".dgf") -> (before substring=→"String Control 3":string)  [unwired: 1 in, 3 out]
            n2901 = Match Pattern(string=w3628, regular expression=".dgf" ("substring (\"\")")) -> (before substring=w3639:string)  [unwired: 1 in, 3 out]
            n2902 = Concatenate Strings(w3639, ".duf" ("Substring")) -> (w3636:string)
            n2903 = String To Path(string=w3636) -> (path=w3634:path)
            n2904 = call <vilib>:"Read Characters From File.vi"("file path (dialog if empty)"=w3634, "start of read offset (chars.:0)"=60 ("start of read offset (chars.: 0)")) -> ("character string"=→"String Control 4":string)  [unwired: 4 in, 3 out]
          }
        }
        n2905 = case shown="True" "OPEN 3" {
          frame False {
          }
          frame True {
            (unwired) 0  # existing file
            w3660 = "Choose a datalog file to open"  # prompt
            n2906 = local write "OPEN 3"(FALSE ("OPEN 1")) -> ()
            n2907 = String To Path(string="C:\\LAB-IQ\\Data\\") -> (path=w3645:path)
            n2908 = File Dialog(6:"*.dgf" ("pattern"), 7:w3660, 11:w3645) -> (0:w3643:errorcluster, 3:w3651:path)  [unwired: 4 in, 2 out]
            n2909 = Unbundle(w3643) -> ()  [unwired: 3 out]
            n2910 = Strip Path(path=w3651) -> (name=w3649:string)  [unwired: 1 out]
            n2911 = Path To String(path=w3651) -> (string=w3646:string)
            "string1 3" <- w3646
            n2912 = Match Pattern(string=w3649, regular expression=".dgf") -> (before substring=→"String Control 5":string)  [unwired: 1 in, 3 out]
            n2913 = Match Pattern(string=w3646, regular expression=".dgf" ("substring (\"\")")) -> (before substring=w3656:string)  [unwired: 1 in, 3 out]
            n2914 = Concatenate Strings(w3656, ".duf" ("Substring")) -> (w3653:string)
            n2915 = String To Path(string=w3653) -> (path=w3657:path)
            n2916 = call <vilib>:"Read Characters From File.vi"("file path (dialog if empty)"=w3657, "start of read offset (chars.:0)"=60 ("start of read offset (chars.: 0)")) -> ("character string"=→"String Control 6":string)  [unwired: 4 in, 3 out]
          }
        }
        n2917 = case shown="True" "OPEN 4" {
          frame False {
          }
          frame True {
            (unwired) 0  # existing file
            w3678 = "Choose a datalog file to open"  # prompt
            n2918 = local write "OPEN 4"(FALSE ("OPEN 1")) -> ()
            n2919 = String To Path(string="C:\\LAB-IQ\\Data\\") -> (path=w3663:path)
            n2920 = File Dialog(6:"*.dgf" ("pattern"), 7:w3678, 11:w3663) -> (0:w3661:errorcluster, 3:w3669:path)  [unwired: 4 in, 2 out]
            n2921 = Unbundle(w3661) -> ()  [unwired: 3 out]
            n2922 = Strip Path(path=w3669) -> (name=w3667:string)  [unwired: 1 out]
            n2923 = Path To String(path=w3669) -> (string=w3664:string)
            "string1 4" <- w3664
            n2924 = Match Pattern(string=w3667, regular expression=".dgf") -> (before substring=→"String Control 7":string)  [unwired: 1 in, 3 out]
            n2925 = Match Pattern(string=w3664, regular expression=".dgf" ("substring (\"\")")) -> (before substring=w3674:string)  [unwired: 1 in, 3 out]
            n2926 = Concatenate Strings(w3674, ".duf" ("Substring")) -> (w3671:string)
            n2927 = String To Path(string=w3671) -> (path=w3675:path)
            n2928 = call <vilib>:"Read Characters From File.vi"("file path (dialog if empty)"=w3675, "start of read offset (chars.:0)"=60 ("start of read offset (chars.: 0)")) -> ("character string"=→"String Control 8":string)  [unwired: 4 in, 3 out]
          }
        }
      }
      frame "About" {
        # "Elapsed time\ncof\nstroke\nmean pos\nTemp\nHumidity"
        n2929 = disable-structure shown="Disabled" {
          frame Disabled {
            n2930 = case shown="True" "Export" {
              frame False {
              }
              frame True {
                w3700 = "                                      " ("string")
                w3702 = "\r"
                (unwired) i16 6 ("width (-)")
                w3779 = "\r"
                w3711 = "\r"
                n2931 = local write "Export"(FALSE ("Export")) -> ()
                n2932 = local read "String 29"() -> (w3748:string)
                n2933 = local read "String 34"() -> (w3736:string)
                n2934 = local read "String 35"() -> (w3731:string)
                n2935 = local read "String 37"() -> (w3727:string)
                n2936 = local read "String 36"() -> (w3724:string)
                n2937 = local read "String 38"() -> (w3721:string)
                n2938 = local read "String 39"() -> (w3718:string)
                n2939 = Match Pattern(string=w3748, regular expression=".dwm") -> (before substring=w3744:string)  [unwired: 1 in, 3 out]
                "before substring" <- w3744
                n2940 = local read "S 38"() -> (w3739:string)
                n2941 = local read "S 39"() -> (w3732:string)
                n2942 = local read "Temperature before test 2"() -> (w3768:dbl)
                n2943 = local read "Temperature after test 2"() -> (w3773:dbl)
                n2944 = local read "Humidity before test 2"() -> (w3754:dbl)
                n2945 = local read "Humidity after test 2"() -> (w3769:dbl)
                n2946 = local read "MWSD 2"() -> (w3765:dbl)
                n2947 = local read "WS1.4 2"() -> (w3781:dbl)
                n2948 = local read "HCF 2"() -> (w3777:dbl)
                n2949 = local read "AVP 2"() -> (w3766:dbl)
                n2950 = Concatenate Strings("1," ("string"), w3739) -> (w3738:string)
                n2951 = Concatenate Strings("2," ("string"), w3736) -> (w3735:string)
                n2952 = Concatenate Strings("3," ("string"), w3732) -> (w3734:string)
                n2953 = Concatenate Strings("4," ("string"), w3731) -> (w3730:string)
                n2954 = Concatenate Strings("5," ("string"), w3727) -> (w3728:string)
                n2955 = Concatenate Strings("6," ("string"), w3724) -> (w3725:string)
                n2956 = Concatenate Strings("7," ("string"), w3721) -> (w3722:string)
                n2957 = Concatenate Strings("8," ("string"), w3718) -> (w3719:string)
                n2958 = local read "Sample ID"() -> (w3786:string)
                n2959 = case shown="\"xlx\"" "Select File Type" {
                  tunnel: w3744 -> [w3789 w3791 w3793]
                  tunnel: [w3787 w3792 w3794] -> w3743
                  frame "xlx" {
                    n2960 = Concatenate Strings(w3789, ".xls" ("string")) -> (w3787:string)
                  }
                  frame "csv" {
                    n2961 = Concatenate Strings(w3791, ".csv" ("string")) -> (w3792:string)
                  }
                  frame "txt" {
                    n2962 = Concatenate Strings(w3793, ".txt" ("string")) -> (w3794:string)
                  }
                }
                n2963 = local read "Test Date"() -> (w3785:string)
                n2964 = local read "String 45"() -> (w3699:string)
                n2965 = local read "String 31"() -> (w3784:string)
                n2966 = local read "String 32"() -> (w3783:string)
                n2967 = local read "TITTLE"() -> (w3707:string)
                n2968 = Number To Fractional String(number=w3754, width (-)=i16 6, precision (6)=i16 2) -> (F-format string=w3753:string)  [unwired: 1 in]
                n2969 = Number To Fractional String(number=w3768, width (-)=i16 6, precision (6)=i16 2) -> (F-format string=w3774:string)  [unwired: 1 in]
                n2970 = Number To Fractional String(number=w3769, width (-)=i16 6, precision (6)=i16 2) -> (F-format string=w3767:string)  [unwired: 1 in]
                n2971 = Number To Fractional String(number=w3773, width (-)=i16 6, precision (6)=i16 2) -> (F-format string=w3772:string)  [unwired: 1 in]
                n2972 = Number To Fractional String(number=w3765, width (-)=i16 6, precision (6)=i16 2) -> (F-format string=w3763:string)  [unwired: 1 in]
                n2973 = Number To Fractional String(number=w3766, width (-)=i16 6, precision (6)=i16 2) -> (F-format string=w3764:string)  [unwired: 1 in]
                n2974 = Number To Fractional String(number=w3777, width (-)=i16 6, precision (6)=i16 2) -> (F-format string=w3778:string)  [unwired: 1 in]
                n2975 = Number To Fractional String(number=w3781, precision (6)=i16 2) -> (F-format string=w3782:string)  [unwired: 2 in]
                n2976 = local read "s.NO"() -> (w3701:string)
                n2977 = Concatenate Strings("=" ("string"), w3707) -> (w3706:string)
                n2978 = Concatenate Strings("S.No," ("string"), "                                       Parameters" ("string")) -> (w3712:string)
                n2979 = Concatenate Strings(w3779, w3738, w3753, w3779, w3735, w3774, w3779, w3734, w3767, w3779, w3730, w3772, w3779, w3728, w3763, w3779, w3725, w3764, w3779, w3722, w3778, w3779, w3719, w3782) -> (w3741:string)
                n2980 = Concatenate Strings(w3711, "," ("string"), w3699, w3701, w3700, w3783, w3786, w3700, w3784, w3785, w3711) -> (w3709:string)
                n2981 = local read "Tested by"() -> (w3715:string)
                n2982 = local read "String 33"() -> (w3716:string)
                n2983 = Concatenate Strings("," ("string"), "                                                                             " ("string")) -> (w3704:string)
                n2984 = Concatenate Strings(w3706, w3702, w3709, w3702, w3712, w3741, w3702, w3704, w3716, w3715) -> (→"export":string)
                n2985 = String To Path(string=w3743) -> (path=w3750:path)
                n2986 = local read "export"() -> (w3745:string)
                n2987 = call <vilib>:"Write Characters To File.vi"("append to file? (new file:F)"=FALSE, "character string"=w3745, "file path (dialog if empty)"=w3750) -> ()  [unwired: 2 in, 1 out]
              }
            }
          }
          frame Enabled {
          }
        }
        n2988 = case shown="True" "OK Button 17" {
          frame False {
          }
          frame True {
            (unwired) 0  # existing file
            w4003 = "Choose a datalog file to open"  # prompt
            n2989 = local write "OK Button 17"(FALSE ("OK Button 17")) -> ()
            n2990 = local read "String"() -> (w3998:string)
            n2991 = String To Path(string=w3998) -> (path=w3999:path)
            n2992 = File Dialog(6:"*.duf" ("pattern"), 7:w4003, 11:w3999) -> (0:w3990:errorcluster, 3:w4009:path)  [unwired: 4 in, 2 out]
            n2993 = Unbundle(w3990) -> ()  [unwired: 3 out]
            n2994 = Open/Create/Replace File "Open File"(file path (use dialog)=w4009) -> (refnum out=w4001:refnum<file>)  [unwired: 5 in, 2 out]
            n2995 = Strip Path(path=w4009) -> (name=w4007:string)  [unwired: 1 out]
            n2996 = Path To String(path=w4009) -> (string=w3992:string)
            n2997 = while {
              tunnel: w4001 -> [w4013]
              i -> [w4010]
              stop <- w4011 continue-if-true
              (unwired) TRUE ("line mode (F)")
              n2998 = Read from Text File "Read File"(file (use dialog)=w4013) -> (text=w4012:string)  [unwired: 3 in, 3 out]
              n2999 = local write "Numeric 16"(w4010) -> ()
              n3000 = String Length(string=w4012) -> (length=w4015:i32)
              n3001 = Greater?(x=w4015, y=1) -> (0:w4011:bool)
            }
            n3002 = local write "String 29"(w3992) -> ()
            n3003 = Search and Replace String(input string=w3992, search string=".duf", replace string=".dgf" ("replace string (\"\")")) -> (result string=→"String Indicator 4":string)  [unwired: 5 in, 3 out]
            n3004 = Match Pattern(string=w4007, regular expression=".dwm") -> (before substring=w3991:string)  [unwired: 1 in, 3 out]
            "String Indicator" <- w3991
            n3005 = Match Pattern(string=w3992, regular expression=".dwm" ("substring (\"\")")) -> (before substring=w3993:string)  [unwired: 1 in, 3 out]
            "String Indicator 3" <- w3993
            n3006 = local write "TITTLE 2"(w3991) -> ()
            n3007 = String To Path(string=w3993) -> (path=w4000:path)
            "path" <- w4000
            n3008 = call <vilib>:"Read Characters From File.vi"("file path (dialog if empty)"=w4000, "start of read offset (chars.:0)"=60 ("start of read offset (chars.: 0)")) -> ("character string"=→"String Indicator 2":string)  [unwired: 4 in, 3 out]
          }
        }
        n3009 = call <vilib>:"Query Available Printers.vi"() -> ("system configured printers"=w3692:string[])  [unwired: 9 in, 2 out]
        "System Configured Printers 2" <- w3692
        n3010 = local read "OK Button 16"() -> (w3689:bool)
        n3011 = case shown="True" "OK Button 16" {
          frame False {
          }
          frame True {
            n3012 = stacked-sequence {
              frame #0 {
                n3013 = local read "Numeric 16"() -> (w4017:i32)
                n3014 = local write "Numeric 10"(w4017) -> ()
              }
              frame #1 {
                n3015 = local read "S.NO"() -> (→"s.NO":string)
                n3016 = local read "String 29"() -> (w4021:string)
                n3017 = String To Path(string=w4021) -> (path=w4020:path)
                n3018 = Open/Create/Replace File "Open File"(file path (use dialog)=w4020) -> (refnum out=w4022:refnum<file>)  [unwired: 5 in, 2 out]
                n3019 = for {
                  N: 16 -> [_]
                  tunnel: w4022 -> [w4029]
                  i -> [w4025]
                  (unwired) TRUE ("line mode (F)")
                  n3020 = Read from Text File "Read File"(file (use dialog)=w4029) -> (text=w4023:string)  [unwired: 3 in, 3 out]
                  n3021 = Match Pattern(string=w4023, regular expression="(") -> (after substring=w4028:string)  [unwired: 1 in, 3 out]
                  n3022 = Match Pattern(string=w4028, regular expression=")") -> (before substring=w4024:string)  [unwired: 1 in, 3 out]
                  n3023 = case shown="1" w4025 {
                    tunnel: w4024 -> [w4030 w4031 _ _ w4032 w4033 w4034 w4036 w4038 w4040 w4042 w4044 w4046 w4048 _]
                    tunnel: w4023 -> [_ _ _ _ _ _ _ _ _ _ _ _ _ _ _]
                    frame 0 {
                      "TITTLE" <- w4030
                    }
                    frame 1 {
                      "Sample ID" <- w4031
                    }
                    frame 2 {
                    }
                    frame 3 {
                    }
                    frame 4 {
                      "Test Date" <- w4032
                    }
                    frame 5 {
                      "Tested by" <- w4033
                    }
                    frame 6 {
                      n3024 = Fract/Exp String To Number(string=w4034) -> (number=→"Humidity before test 2":dbl)  [unwired: 3 in, 1 out]
                    }
                    frame 7 {
                      n3025 = Fract/Exp String To Number(string=w4036) -> (number=→"Temperature before test 2":dbl)  [unwired: 3 in, 1 out]
                    }
                    frame 8 {
                      n3026 = Fract/Exp String To Number(string=w4038) -> (number=→"Humidity after test 2":dbl)  [unwired: 3 in, 1 out]
                    }
                    frame 9 {
                      n3027 = Fract/Exp String To Number(string=w4040) -> (number=→"Temperature after test 2":dbl)  [unwired: 3 in, 1 out]
                    }
                    frame 10 {
                      n3028 = Fract/Exp String To Number(string=w4042) -> (number=→"MWSD 2":dbl)  [unwired: 3 in, 1 out]
                    }
                    frame 11 {
                      n3029 = Fract/Exp String To Number(string=w4044) -> (number=→"AVP 2":dbl)  [unwired: 3 in, 1 out]
                    }
                    frame 12 {
                      n3030 = Fract/Exp String To Number(string=w4046) -> (number=→"HCF 2":dbl)  [unwired: 3 in, 1 out]
                    }
                    frame 13 {
                      n3031 = Fract/Exp String To Number(string=w4048) -> (number=→"WS1.4 2":dbl)  [unwired: 3 in, 1 out]
                    }
                    frame 14, Default {
                    }
                  }
                }
              }
              frame #2 {
              }
            }
            n3032 = local write "OK Button 16"(FALSE ("OK Button 13")) -> ()
          }
        }
        n3033 = Index Array(array=w3692, index="Select Printer 3") -> (element=w3694:string)
        "Selected Printer" <- w3694
        n3034 = case shown="True" w3689 {
          frame False {
          }
          frame True {
            n3035 = flat-sequence {
              frame #0 {
              }
              frame #1 {
                n3036 = Wait (ms)(milliseconds to wait=u32 100) -> ()  [unwired: 1 out]
              }
              frame #2 {
                n3037 = local write "OK Button 16"(FALSE ("Print 3")) -> ()
              }
            }
          }
        }
        n3038 = case shown="True" "Print" {
          tunnel: w3694 -> [_ w3986]
          frame False {
          }
          frame True {
            (unwired) i16 6 ("width (-)")
            (unwired) "TESTED BY : "
            (unwired) "TESTED DATE :"
            (unwired) "SAMPLE ID : "
            (unwired) "SAMPLE DESIGN : "
            w3944 = "\r"
            w3961 = "\r"
            # "add image"
            n3039 = local read "Sample ID"() -> (w3934:string)
            n3040 = local read "Tested by"() -> (w3937:string)
            n3041 = local read "String 34"() -> (w3924:string)
            n3042 = local read "String 45"() -> (w3904:string)
            n3043 = local read "String 35"() -> (w3919:string)
            n3044 = local read "String 37"() -> (w3917:string)
            n3045 = local read "String 32"() -> (w3939:string)
            n3046 = local read "String 36"() -> (w3914:string)
            n3047 = local read "String 31"() -> (w3938:string)
            n3048 = local read "Test Date"() -> (w3935:string)
            n3049 = local read "String 33"() -> (w3940:string)
            n3050 = local read "String 38"() -> (w3910:string)
            n3051 = local read "String 39"() -> (w3907:string)
            n3052 = local write "Print"(FALSE ("Print FF")) -> ()
            n3053 = local read "S 39"() -> (w3922:string)
            n3054 = local read "S 38"() -> (w3929:string)
            n3055 = local read "Temperature before test 2"() -> (w3960:dbl)
            n3056 = local read "Temperature after test 2"() -> (w3950:dbl)
            n3057 = local read "Humidity before test 2"() -> (w3975:dbl)
            n3058 = local read "Humidity after test 2"() -> (w3959:dbl)
            n3059 = local read "MWSD 2"() -> (w3964:dbl)
